vi "Write.vi"(8 "error in (no error)":errorcluster, 10 "element":variant, 11 "NetworkStreamWriter in":refnum<class "NetworkStreamWriter.lvclass">) -> (0 "error out":errorcluster, 3 "NetworkStreamWriter out":refnum<class "NetworkStreamWriter.lvclass">)   [LabVIEW 2011, in "NetworkStreamWriter.lvclass"]
doc: "Returns the requested value (either the next element available in the buffer or the most recent element). If there are no elements available in the queue, this VI will return the last valid value it returned.\n\nWrites the requested value to the internal queue, which will be sent across the network asynchronously by the WriterDaemon."
uses:
  NetworkStreamWriter.lvclass
  NetworkStreamWriter.lvclass/NetworkStreamWriter.ctl
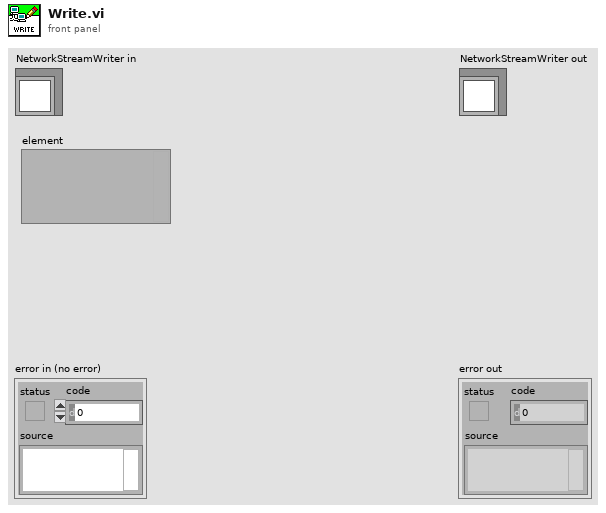
[diagram p1: front panel]
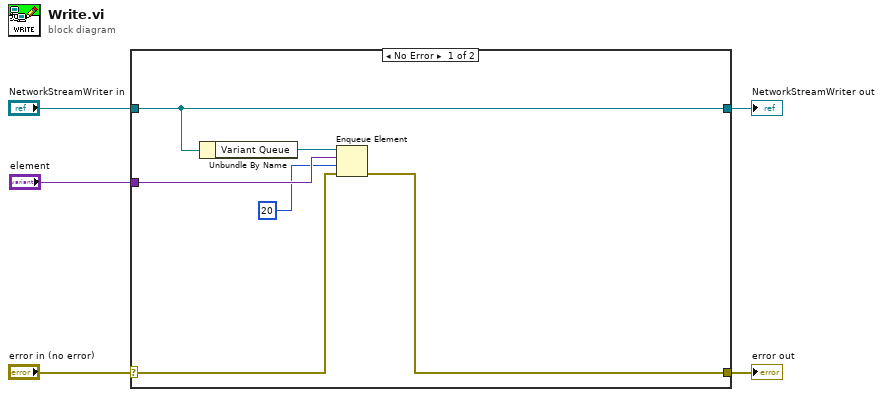
[diagram p0: block diagram]
diagram:
  n1 = case shown="No Error" "error in (no error)" {
    selector: "error in (no error)" -> [w8 w13]
    tunnel: [w6 w13] -> w4
    tunnel: [w11 w12] -> w2
    tunnel: "NetworkStreamWriter in" -> [w11 w12]
    tunnel: "element" -> [w9 _]
    frame No Error {
      n2 = Unbundle By Name(w11) -> ("Variant Queue"=w10:refnum<queue>)
      n3 = Enqueue Element(queue=w10, element=w9, timeout in ms (-1)=20, error in (no error)=w8) -> (error out=w6:errorcluster)  [unwired: 2 out]
    }
    frame Error {
    }
  }
  "error out" <- w4
  "NetworkStreamWriter out" <- w2
